vi "chanDescQSB.vi"(1 "dimensions":i64[](array[numeric])=[1399090569999999999, -1], 2 "values":T1(array[cluster])=[{"chanDescs"=[{"name"="E_Chan_1", "active"=1}, {"name"="E_Chan_2", "active"=1}, {"name"="E_Chan_3", "active"=1}, {"name"="E_Chan_4", "active"=1}, {"name"="E_Chan_5", "active"=1}, {"name"="E_Chan_6", "active"=1}, {"name"="E_Chan_7", "active"=1}, {"name"="E_Chan_8", "active"=1}, {"name"="E_Chan_9", "active"=1}, {"name"="E_Chan_10", "active"=1}, {"name"="E_Chan_11", "active"=1}, {"name"="E_Chan_12", "active"=1}, {"name"="E_Chan_13", "active"=1}, {"name"="E_Chan_14", "active"=1}, {"name"="E_Chan_15", "active"=1}, {"name"="E_Chan_16", "active"=1}, {"name"="E_Chan_17", "active"=1}, {"name"="E_Chan_18", "active"=1}, {"name"="E_Chan_19", "active"=1}, {"name"="E_Chan_20", "active"=1}, {"name"="E_Chan_21", "active"=1}, {"name"="E_Chan_22", "active"=1}, {"name"="E_Chan_23", "active"=1}, {"name"="E_Chan_24", "active"=1}, {"name"="E_Chan_25", "active"=1}, {"name"="E_Chan_26", "active"=1}, {"name"="E_Chan_27", "active"=1}, {"name"="E_Chan_28", "active"=1}, {"name"="E_Chan_29", "active"=1}, {"name"="E_Chan_30", "active"=1}, {"name"="E_Chan_31", "active"=1}, {"name"="E_Chan_32", "active"=1}, {"name"="E_Chan_33", "active"=1}, {"name"="E_Chan_34", "active"=1}, {"name"="E_Chan_35", "active"=1}, {"name"="E_Chan_36", "active"=1}, {"name"="E_Chan_37", "active"=1}, {"name"="E_Chan_38", "active"=1}, {"name"="E_Chan_39", "active"=1}, {"name"="E_Chan_40", "active"=1}, {"name"="E_Chan_41", "active"=1}, {"name"="E_Chan_42", "active"=1}, {"name"="E_Chan_43", "active"=1}, {"name"="E_Chan_44", "active"=1}, {"name"="E_Chan_45", "active"=1}, {"name"="E_Chan_46", "active"=1}, {"name"="E_Chan_47", "active"=1}, {"name"="E_Chan_48", "active"=1}, {"name"="E_Chan_49", "active"=1}, {"name"="E_Chan_50", "active"=1}, {"name"="E_Chan_51", "active"=1}, {"name"="E_Chan_52", "active"=1}, {"name"="E_Chan_53", "active"=1}, {"name"="E_Chan_54", "active"=1}, {"name"="E_Chan_55", "active"=1}, {"name"="E_Chan_56", "active"=1}, {"name"="E_Chan_57", "active"=1}, {"name"="E_Chan_58", "active"=1}, {"name"="E_Chan_59", "active"=1}, {"name"="E_Chan_60", "active"=1}, {"name"="E_Chan_61", "active"=1}, {"name"="E_Chan_62", "active"=1}, {"name"="E_Chan_63", "active"=1}, {"name"="E_Chan_64", "active"=1}, {"name"="E_Chan_65", "active"=1}, {"name"="E_Chan_66", "active"=1}, {"name"="E_Chan_67", "active"=1}, {"name"="E_Chan_68", "active"=1}, {"name"="E_Chan_69", "active"=1}, {"name"="E_Chan_70", "active"=1}, {"name"="E_Chan_71", "active"=1}, {"name"="E_Chan_72", "active"=1}, {"name"="E_Chan_73", "active"=1}, {"name"="E_Chan_74", "active"=1}, {"name"="E_Chan_75", "active"=1}, {"name"="E_Chan_76", "active"=1}, {"name"="E_Chan_77", "active"=1}, {"name"="E_Chan_78", "active"=1}, {"name"="E_Chan_79", "active"=1}, {"name"="E_Chan_80", "active"=1}, {"name"="E_Chan_81", "active"=1}, {"name"="E_Chan_82", "active"=1}, {"name"="E_Chan_83", "active"=1}, {"name"="E_Chan_84", "active"=1}, {"name"="E_Chan_85", "active"=1}, {"name"="E_Chan_86", "active"=1}, {"name"="E_Chan_87", "active"=1}, {"name"="E_Chan_88", "active"=1}, {"name"="E_Chan_89", "active"=1}, {"name"="E_Chan_90", "active"=1}, {"name"="E_Chan_91", "active"=1}, {"name"="E_Chan_92", "active"=1}, {"name"="E_Chan_93", "active"=1}, {"name"="E_Chan_94", "active"=1}, {"name"="E_Chan_95", "active"=1}, {"name"="E_Chan_96", "active"=1}, {"name"="E_Chan_97", "active"=1}, {"name"="E_Chan_98", "active"=1}, {"name"="E_Chan_99", "active"=1}, {"name"="E_Chan_100", "active"=1}, {"name"="E_Chan_101", "active"=1}, {"name"="E_Chan_102", "active"=1}, {"name"="E_Chan_103", "active"=1}, {"name"="E_Chan_104", "active"=1}, {"name"="E_Chan_105", "active"=1}, {"name"="E_Chan_106", "active"=1}, {"name"="E_Chan_107", "active"=1}, {"name"="E_Chan_108", "active"=1}, {"name"="E_Chan_109", "active"=1}, {"name"="E_Chan_110", "active"=1}, {"name"="E_Chan_111", "active"=1}, {"name"="E_Chan_112", "active"=1}, {"name"="E_Chan_113", "active"=1}, {"name"="E_Chan_114", "active"=1}, {"name"="E_Chan_115", "active"=1}, {"name"="E_Chan_116", "active"=1}, {"name"="E_Chan_117", "active"=1}, {"name"="E_Chan_118", "active"=1}, {"name"="E_Chan_119", "active"=1}, {"name"="E_Chan_120", "active"=1}, {"name"="E_Chan_121", "active"=1}, {"name"="E_Chan_122", "active"=1}, {"name"="E_Chan_123", "active"=1}, {"name"="E_Chan_124", "active"=1}, {"name"="E_Chan_125", "active"=1}, {"name"="E_Chan_126", "active"=1}, {"name"="E_Chan_127", "active"=1}, {"name"="E_Chan_128", "active"=1}]}], 3 "label":string="parms") -> (0 "JSON string":string="{\"label\":\"parms\",\"values\":[{\"chanDescs\":[{\"name\":\"HBCm_U30_01\",\"active\":1},{\"name\":\"HBCm_U30_02\",\"active\":1},{\"name\":\"HBCm_U30_03\",\"active\":1},{\"name\":\"HBCm_U30_04\",\"active\":1},{\"name\":\"HBCm_U30_05\",\"active\":1},{\"name\":\"HBCm_U30_06\",\"active\":1},{\"name\":\"HBCm_U30_07\",\"active\":1},{\"name\":\"HBCm_U30_08\",\"active\":1},{\"name\":\"HBCm_U30_09\",\"active\":1},{\"name\":\"HBCm_U30_10\",\"active\":1},{\"name\":\"HBCm_U30_11\",\"active\":1},{\"name\":\"HBCm_U30_12\",\"active\":1},{\"name\":\"HBCm_U30_13\",\"active\":1},{\"name\":\"HBCm_U30_14\",\"active\":1},{\"name\":\"HBCm_U30_15\",\"active\":1},{\"name\":\"HBCm_U30_16\",\"active\":1},{\"name\":\"HBCm_U30_17\",\"active\":1},{\"name\":\"HBCm_U30_18\",\"active\":1},{\"name\":\"HBCm_U30_19\",\"active\":1},{\"name\":\"HBCm_U30_20\",\"active\":1},{\"name\":\"HBCm_U30_21\",\"active\":1},{\"name\":\"HBCm_U30_22\",\"active\":1},{\"name\":\"HBCm_U30_23\",\"active\":1},{\"name\":\"HBCm_U30_24\",\"active\":1},{\"name\":\"HBCm_U30_25\",\"active\":1},{\"name\":\"HBCm_U30_26\",\"active\":1},{\"name\":\"HBCm_U30_27\",\"active\":1},{\"name\":\"HBCm_U30_28\",\"active\":1},{\"name\":\"HBCm_U30_29\",\"active\":1},{\"name\":\"HBCm_U30_30\",\"active\":1},{\"name\":\"HBCm_U30_31\",\"active\":1},{\"name\":\"HBCm_U30_32\",\"active\":1},{\"name\":\"HBCm_V21_01\",\"active\":1},{\"name\":\"HBCm_V21_02\",\"active\":1},{\"name\":\"HBCm_V21_03\",\"active\":1},{\"name\":\"HBCm_V21_04\",\"active\":1},{\"name\":\"HBCm_V21_05\",\"active\":1},{\"name\":\"HBCm_V21_06\",\"active\":1},{\"name\":\"HBCm_V21_07\",\"active\":1},{\"name\":\"HBCm_V21_08\",\"active\":1},{\"name\":\"HBCm_V21_09\",\"active\":1},{\"name\":\"HBCm_V21_10\",\"active\":1},{\"name\":\"HBCm_V21_11\",\"active\":1},{\"name\":\"HBCm_V21_12\",\"active\":1},{\"name\":\"HBCm_V21_13\",\"active\":1},{\"name\":\"HBCm_V21_14\",\"active\":1},{\"name\":\"HBCm_V21_15\",\"active\":1},{\"name\":\"HBCm_V21_16\",\"active\":1},{\"name\":\"HBCm_V21_17\",\"active\":1},{\"name\":\"HBCm_V21_18\",\"active\":1},{\"name\":\"HBCm_V21_19\",\"active\":1},{\"name\":\"HBCm_V21_20\",\"active\":1},{\"name\":\"HBCm_V21_21\",\"active\":1},{\"name\":\"HBCm_V21_22\",\"active\":1},{\"name\":\"HBCm_V21_23\",\"active\":1},{\"name\":\"HBCm_V21_24\",\"active\":1},{\"name\":\"HBCm_V21_25\",\"active\":1},{\"name\":\"HBCm_V21_26\",\"active\":1},{\"name\":\"HBCm_V21_27\",\"active\":1},{\"name\":\"HBCm_V21_28\",\"active\":1},{\"name\":\"HBCm_V21_29\",\"active\":1},{\"name\":\"HBCm_V21_30\",\"active\":1},{\"name\":\"HBCm_V21_31\",\"active\":1},{\"name\":\"HBCm_V21_32\",\"active\":1},{\"name\":\"HBCm_V21_33\",\"active\":1},{\"name\":\"HBCm_V21_34\",\"active\":1},{\"name\":\"HBCm_V21_35\",\"active\":1},{\"name\":\"HBCm_V21_36\",\"active\":1},{\"name\":\"HBCm_V21_37\",\"active\":1},{\"name\":\"HBCm_V21_38\",\"active\":1},{\"name\":\"HBCm_V21_39\",\"active\":1},{\"name\":\"HBCm_V21_40\",\"active\":1},{\"name\":\"VBCs_V21_01\",\"active\":1},{\"name\":\"VBCs_V21_02\",\"active\":1},{\"name\":\"VBCs_V21_03\",\"active\":1},{\"name\":\"VBCs_V21_04\",\"active\":1},{\"name\":\"VBCs_V21_05\",\"active\":1},{\"name\":\"VBCs_V21_06\",\"active\":1},{\"name\":\"VBCs_V21_08\",\"active\":1},{\"name\":\"VBCs_V21_09\",\"active\":0},{\"name\":\"VBCs_V21_01\",\"active\":1},{\"name\":\"VBCs_V21_02\",\"active\":1},{\"name\":\"VBCs_V21_03\",\"active\":1},{\"name\":\"VBCs_V21_04\",\"active\":1},{\"name\":\"VBCs_V21_05\",\"active\":1},{\"name\":\"VBCs_V21_06\",\"active\":1},{\"name\":\"VBCs_V21_07\",\"active\":1},{\"name\":\"VBCs_V21_08\",\"active\":1},{\"name\":\"VBCs_V21_09\",\"active\":1},{\"name\":\"VBCs_V21_09\",\"active\":1},{\"name\":\"VBCs_V21_10\",\"active\":1},{\"name\":\"VBCs_V21_11\",\"active\":1},{\"name\":\"VBCs_V21_12\",\"active\":1},{\"name\":\"VBCs_V21_13\",\"active\":1},{\"name\":\"VBCs_V21_14\",\"active\":1},{\"name\":\"VBCs_V21_15\",\"active\":1}]}],\"dimensions\":[1399090569999999999,-1]}")   [LabVIEW 2014]
panel:
  in  "chanDescs 2":cluster{"name":string, "active":i32}[](array[cluster])=[{"name"="E_Chan_1", "active"=1}, {"name"="E_Chan_2", "active"=1}, {"name"="E_Chan_3", "active"=1}, {"name"="E_Chan_4", "active"=1}, {"name"="E_Chan_5", "active"=1}, {"name"="E_Chan_6", "active"=1}, {"name"="E_Chan_7", "active"=1}, {"name"="E_Chan_8", "active"=1}, {"name"="E_Chan_9", "active"=1}, {"name"="E_Chan_10", "active"=1}, {"name"="E_Chan_11", "active"=1}, {"name"="E_Chan_12", "active"=1}, {"name"="E_Chan_13", "active"=1}, {"name"="E_Chan_14", "active"=1}, {"name"="E_Chan_15", "active"=1}, {"name"="E_Chan_16", "active"=1}, {"name"="E_Chan_17", "active"=1}, {"name"="E_Chan_18", "active"=1}, {"name"="E_Chan_19", "active"=1}, {"name"="E_Chan_20", "active"=1}, {"name"="E_Chan_21", "active"=1}, {"name"="E_Chan_22", "active"=1}, {"name"="E_Chan_23", "active"=1}, {"name"="E_Chan_24", "active"=1}, {"name"="E_Chan_25", "active"=1}, {"name"="E_Chan_26", "active"=1}, {"name"="E_Chan_27", "active"=1}, {"name"="E_Chan_28", "active"=1}, {"name"="E_Chan_29", "active"=1}, {"name"="E_Chan_30", "active"=1}, {"name"="E_Chan_31", "active"=1}, {"name"="E_Chan_32", "active"=1}, {"name"="E_Chan_33", "active"=1}, {"name"="E_Chan_34", "active"=1}, {"name"="E_Chan_35", "active"=1}, {"name"="E_Chan_36", "active"=1}, {"name"="E_Chan_37", "active"=1}, {"name"="E_Chan_38", "active"=1}, {"name"="E_Chan_39", "active"=1}, {"name"="E_Chan_40", "active"=1}, {"name"="E_Chan_41", "active"=1}, {"name"="E_Chan_42", "active"=1}, {"name"="E_Chan_43", "active"=1}, {"name"="E_Chan_44", "active"=1}, {"name"="E_Chan_45", "active"=1}, {"name"="E_Chan_46", "active"=1}, {"name"="E_Chan_47", "active"=1}, {"name"="E_Chan_48", "active"=1}, {"name"="E_Chan_49", "active"=1}, {"name"="E_Chan_50", "active"=1}, {"name"="E_Chan_51", "active"=1}, {"name"="E_Chan_52", "active"=1}, {"name"="E_Chan_53", "active"=1}, {"name"="E_Chan_54", "active"=1}, {"name"="E_Chan_55", "active"=1}, {"name"="E_Chan_56", "active"=1}, {"name"="E_Chan_57", "active"=1}, {"name"="E_Chan_58", "active"=1}, {"name"="E_Chan_59", "active"=1}, {"name"="E_Chan_60", "active"=1}, {"name"="E_Chan_61", "active"=1}, {"name"="E_Chan_62", "active"=1}, {"name"="E_Chan_63", "active"=1}, {"name"="E_Chan_64", "active"=1}, {"name"="E_Chan_65", "active"=1}, {"name"="E_Chan_66", "active"=1}, {"name"="E_Chan_67", "active"=1}, {"name"="E_Chan_68", "active"=1}, {"name"="E_Chan_69", "active"=1}, {"name"="E_Chan_70", "active"=1}, {"name"="E_Chan_71", "active"=1}, {"name"="E_Chan_72", "active"=1}, {"name"="E_Chan_73", "active"=1}, {"name"="E_Chan_74", "active"=1}, {"name"="E_Chan_75", "active"=1}, {"name"="E_Chan_76", "active"=1}, {"name"="E_Chan_77", "active"=1}, {"name"="E_Chan_78", "active"=1}, {"name"="E_Chan_79", "active"=1}, {"name"="E_Chan_80", "active"=1}, {"name"="E_Chan_81", "active"=1}, {"name"="E_Chan_82", "active"=1}, {"name"="E_Chan_83", "active"=1}, {"name"="E_Chan_84", "active"=1}, {"name"="E_Chan_85", "active"=1}, {"name"="E_Chan_86", "active"=1}, {"name"="E_Chan_87", "active"=1}, {"name"="E_Chan_88", "active"=1}, {"name"="E_Chan_89", "active"=1}, {"name"="E_Chan_90", "active"=1}, {"name"="E_Chan_91", "active"=1}, {"name"="E_Chan_92", "active"=1}, {"name"="E_Chan_93", "active"=1}, {"name"="E_Chan_94", "active"=1}, {"name"="E_Chan_95", "active"=1}, {"name"="E_Chan_96", "active"=1}, {"name"="E_Chan_97", "active"=1}, {"name"="E_Chan_98", "active"=1}, {"name"="E_Chan_99", "active"=1}, {"name"="E_Chan_100", "active"=1}, {"name"="E_Chan_101", "active"=1}, {"name"="E_Chan_102", "active"=1}, {"name"="E_Chan_103", "active"=1}, {"name"="E_Chan_104", "active"=1}, {"name"="E_Chan_105", "active"=1}, {"name"="E_Chan_106", "active"=1}, {"name"="E_Chan_107", "active"=1}, {"name"="E_Chan_108", "active"=1}, {"name"="E_Chan_109", "active"=1}, {"name"="E_Chan_110", "active"=1}, {"name"="E_Chan_111", "active"=1}, {"name"="E_Chan_112", "active"=1}, {"name"="E_Chan_113", "active"=1}, {"name"="E_Chan_114", "active"=1}, {"name"="E_Chan_115", "active"=1}, {"name"="E_Chan_116", "active"=1}, {"name"="E_Chan_117", "active"=1}, {"name"="E_Chan_118", "active"=1}, {"name"="E_Chan_119", "active"=1}, {"name"="E_Chan_120", "active"=1}, {"name"="E_Chan_121", "active"=1}, {"name"="E_Chan_122", "active"=1}, {"name"="E_Chan_123", "active"=1}, {"name"="E_Chan_124", "active"=1}, {"name"="E_Chan_125", "active"=1}, {"name"="E_Chan_126", "active"=1}, {"name"="E_Chan_127", "active"=1}, {"name"="E_Chan_128", "active"=1}]
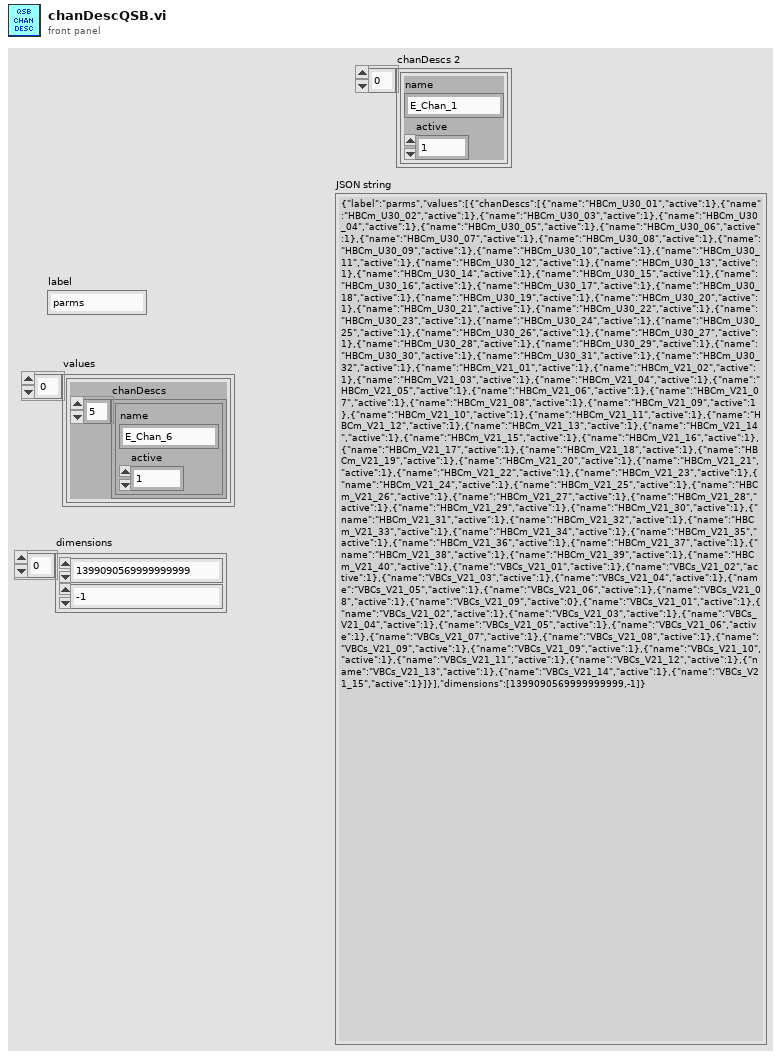
[diagram p1: front panel]
types:
  T1 = cluster{"chanDescs":cluster{"name":string, "active":i32}[]}[]
  T2 = cluster{"label":string, "values":cluster{"chanDescs":cluster{"name":string, "active":i32}[]}[], "dimensions":i64[]}
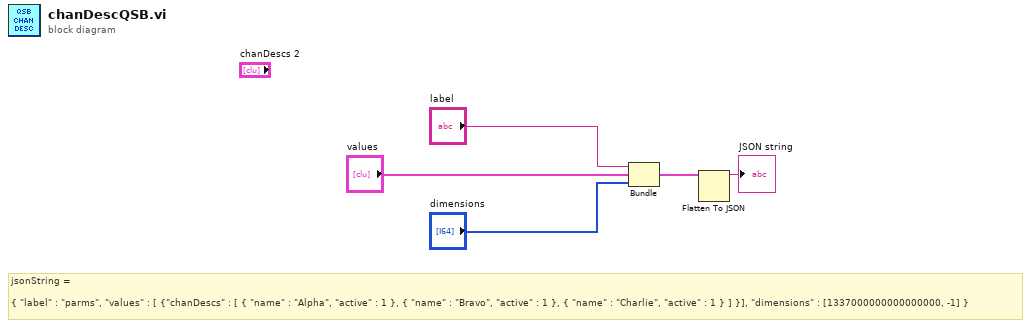
[diagram p0: block diagram]
diagram:
  # "jsonString = \n\n{ \"label\" : \"parms\", \"values\" : [ {\"chanDescs\" : [ { \"name\" : \"Alpha\", \"active\" : 1 }, { \"name\" : \"Bravo\", \"active\" : 1 }, { \"name\" : \"Charlie\", \"active\" : 1 } ] }], \"dimensions\" : [1337000000000000000, -1] }"
  n1 = Bundle("label"="label", "values"="values", "dimensions"="dimensions") -> (w4:T2)  [unwired: 1 in]
  n2 = Flatten To JSON(anything=w4) -> (JSON string=→"JSON string":string)  [unwired: 2 in, 1 out]
